vi "Measurement Logic.vi"() -> ()   [LabVIEW 2021, in "SimpleSwitchDisconnect.lvlib"]
uses:
  SimpleSwitchDisconnect.lvlib
  <vilib>/Plug-In SDKs/Measurements/Measure Call Context/Measure Call Context.lvclass
  Measurement Configuration.ctl
  SimpleSwitch UI/Initialization Behavior.ctl
  Measurement Results.ctl
  <vilib>/Utility/error.llb/DialogType.ctl
  <vilib>/Plug-In SDKs/Clients/Session Management V1/Session Reservation/Session Reservation.lvclass
  Sessions/niSE/NI Session Management niSE.lvlib
  Sessions/niSE/Session Factory/Session Factory.lvclass
  SimpleSwitch UI/SimpleSwitchDisconnect UI.lvlib
panel:
  out "measurement results":T1
  in  "measurement configuration":T2={"pin_name"="Lorem ipsum dolor sit", "Option String (\"\")"="", "Disconnect Specification (\"\")"="", "Initialization Behavior"=enum."Auto"}
  out "measure call context out":refnum<class "Measure Call Context.lvclass">
  in  "measure call context in":refnum<class "Measure Call Context.lvclass">
  out "error out":errorcluster
  in  "error in":errorcluster
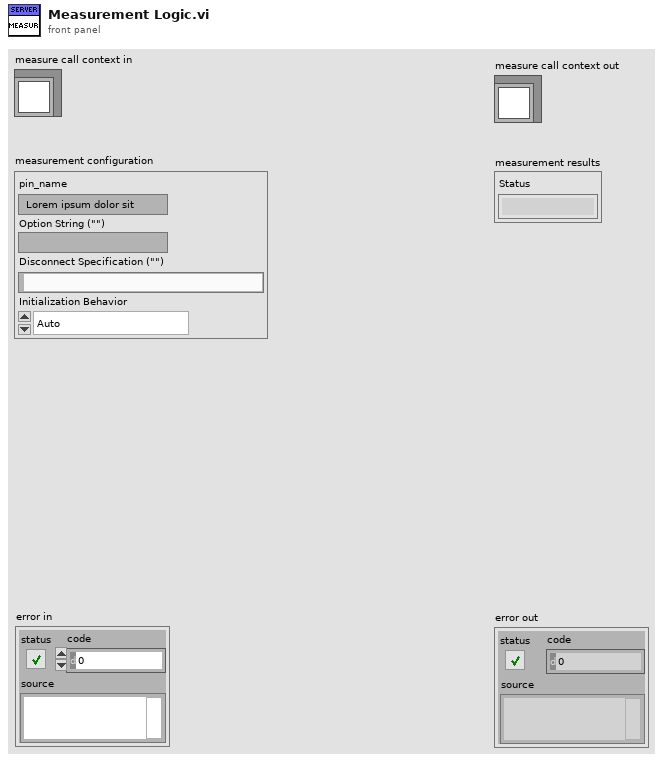
[diagram p1: front panel]
types:
  T1 = typedef "SimpleSwitchDisconnect.lvlib/Measurement Results.ctl" = cluster{"Status":string}
  T2 = typedef "SimpleSwitchDisconnect.lvlib/Measurement Configuration.ctl" = cluster{"pin_name":string, "Option String (\"\")":string, "Disconnect Specification (\"\")":string, "Initialization Behavior":T3}
  T3 = typedef "SimpleSwitchDisconnect UI.lvlib/Initialization Behavior.ctl" = enum32{"Auto", "Initialize and Close", "Attach and Detach", "Initialize and Detach", "Attach and Close"}
  T4 = typedef "DialogType.ctl" = u16
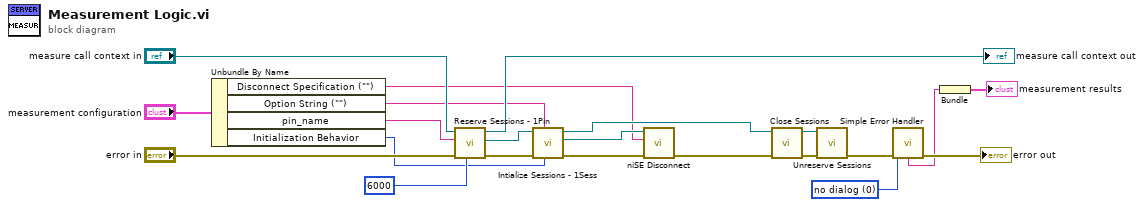
[diagram p0: block diagram]
diagram:
  w4 = T4 0 items=["no dialog", "OK message", "continue or stop message", "OK message + warnings", "continue/stop + warnings"] ("type of dialog (OK msg:1)")
  n1 = Unbundle By Name("measurement configuration") -> ("Disconnect Specification (\"\")"=w7:string, "Option String (\"\")"=w14:string, "pin_name"=w20:string, "Initialization Behavior"=w1:T3)
  n2 = call <vilib>:"Reserve Sessions - 1Pin.vi"("timeout (ms)"=6000, "error in"="error in", "pin or relay name"=w20, "measurement context in"="measure call context in") -> ("error out"=w18:errorcluster, "session reservation out"=w17:refnum<class "Session Reservation.lvclass">, "measurement context out"=→"measure call context out":refnum<class "Measure Call Context.lvclass">)  [unwired: 5 in]
  n3 = call "Intialize Sessions - 1Sess.vi"("initialize and close session behavior"=w1, "option string"=w14, "error in"=w18, "session reservation in"=w17) -> ("error out"=w9:errorcluster, "session"=w8:refnum<class "Session Factory.lvclass">, "session reservation out"=w10:refnum<class "Session Reservation.lvclass">)  [unwired: 5 in]
  n4 = call "niSE Disconnect.vi"("error in (no error)"=w9, "disconnect_specification"=w7, "Session Factory in"=w8) -> ("error out"=w6:errorcluster)  [unwired: 7 in, 1 out]
  n5 = call <vilib>:"Close Sessions.vi"("error in"=w6, "session reservation in"=w10) -> ("error out"=w13:errorcluster, "session reservation out"=w12:refnum<class "Session Reservation.lvclass">)  [unwired: 8 in]
  n6 = call <vilib>:"Unreserve Sessions.vi"("error in"=w13, "session reservation in"=w12) -> ("error out"=w11:errorcluster)  [unwired: 9 in]
  n7 = call <vilib>:"Simple Error Handler.vi"("type of dialog (OK msg:1)"=w4, "error in (no error)"=w11) -> ("error out"=→"error out":errorcluster, "message"=w3:string)  [unwired: 3 in, 3 out]
  n8 = Bundle("message"=w3) -> (→"measurement results":cluster{"message":string})  [unwired: 1 in]
